vi "Discard correct num element.vi"(2 "Read packet dim":u32, 3 "Element Remaing in Queue":u32, 4 "FPGA VI Reference In":refnum<k20>) -> (1 "error out":errorcluster)   [LabVIEW 2014]
doc: "This subVI is used to empty DMA queues. FPGA writes on DMA more speedy than microcontroller read. For this, it's needed to discard a portion of values from DMA for each DMA reading in order to avoid bottleneck."
uses:
  <vilib>/Utility/error.llb/Error Cluster From Error Code.vi
  <vilib>/rvi/errors/niLvFpgaAdjustHostInterfaceError.vi
  <vilib>/rvi/interface/nirviMethod/nirviMethod.xnode
  <vilib>/FPGAPlugInAG/Dynamic/niLvFpga_ReadFifo_Dynamic.vi
  <vilib>/rvi/errors/niLvFpgaMergeErrorWithErrorCode.vi
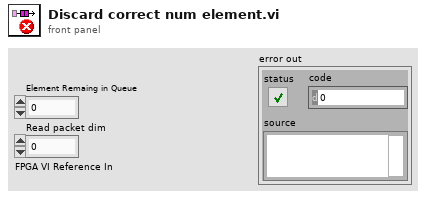
[diagram p1: front panel]
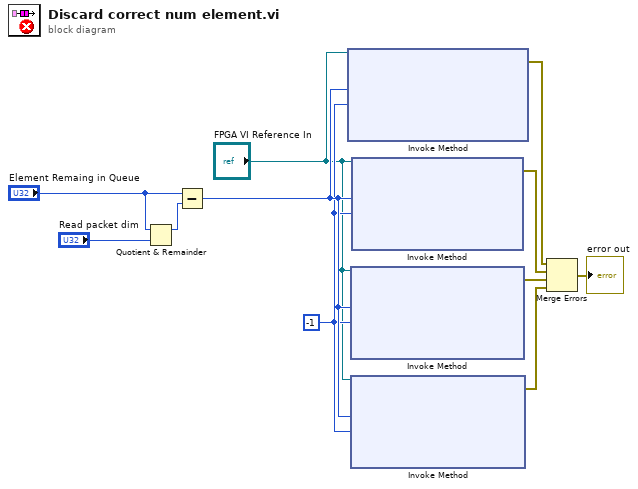
[diagram p0: block diagram]
diagram:
  w7 = -1 ("Timeout (ms)")
  n1 = Quotient & Remainder(x="Element Remaing in Queue", y="Read packet dim") -> (x-y*floor(x/y)=w9:u32)  [unwired: 1 out]
  n2 = Subtract(x="Element Remaing in Queue", y=w9) -> (x-y=w8:u32)
  n3 = xnode "Invoke Method"("FPGA VI Reference In"="FPGA VI Reference In", "Number of Elements"=w8, "Timeout (ms)"=w7) -> ("error out"=w2:errorcluster)  [unwired: 1 in, 3 out]
  n4 = xnode "Invoke Method"("FPGA VI Reference In"="FPGA VI Reference In", "Number of Elements"=w8, "Timeout (ms)"=w7) -> ("error out"=w4:errorcluster)  [unwired: 1 in, 3 out]
  n5 = xnode "Invoke Method"("FPGA VI Reference In"="FPGA VI Reference In", "Number of Elements"=w8, "Timeout (ms)"=w7) -> ("error out"=w5:errorcluster)  [unwired: 1 in, 3 out]
  n6 = xnode "Invoke Method"("FPGA VI Reference In"="FPGA VI Reference In", "Number of Elements"=w8, "Timeout (ms)"=w7) -> ("error out"=w3:errorcluster)  [unwired: 1 in, 3 out]
  n7 = Merge Errors(w2, w3, w4, w5) -> (→"error out":errorcluster)
